vi "Error - Fire.vi"(6 "Data":variant, 8 "error in (no error)":errorcluster, 9 "Error Source":T1, 10 "Error Type":T2, 11 "View Model":T3) -> (0 "error out":errorcluster, 3 "View Model":T3)   [LabVIEW 2017]
doc: "Generate user Event for Error event"
uses:
  View Model/Controls/View Model.ctl
  View Model/Controls/Shared Model.ctl
  Controls/Error Model.ctl
  Controls/Error Data.ctl
  Controls/Error Type.ctl
  Controls/Error Source.ctl
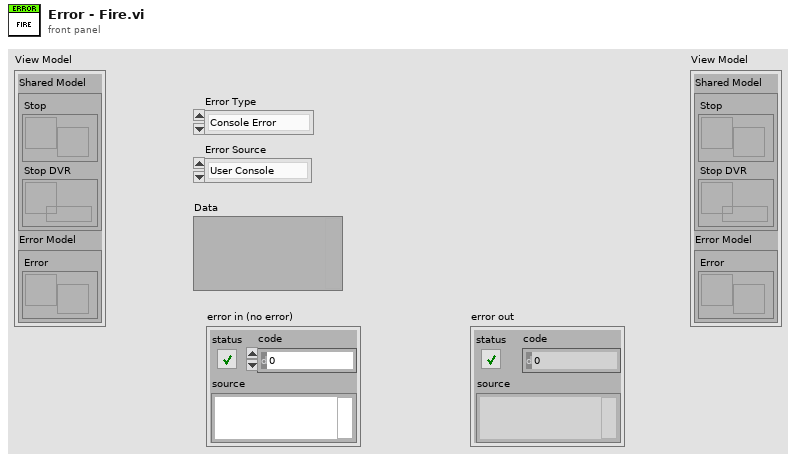
[diagram p1: front panel]
types:
  T1 = typedef "Error Source.ctl" = enum16{"User Console", "Display Console", "Sensor Interface"}
  T2 = typedef "Error Type.ctl" = enum16{"Console Error", "Sensor Interface IO Error", "Process Step Error"}
  T3 = typedef "View Model.ctl" = cluster{"Shared Model":T4, "Error Model":T5}
  T4 = typedef "Shared Model.ctl" = cluster{"Stop":refnum<user-event>, "Stop DVR":refnum<data-value>}
  T5 = typedef "Error Model.ctl" = cluster{"Error":refnum<user-event>}
  T6 = typedef "Error Data.ctl" = cluster{"Error Type":T2, "Error Source":T1, "Data":variant}
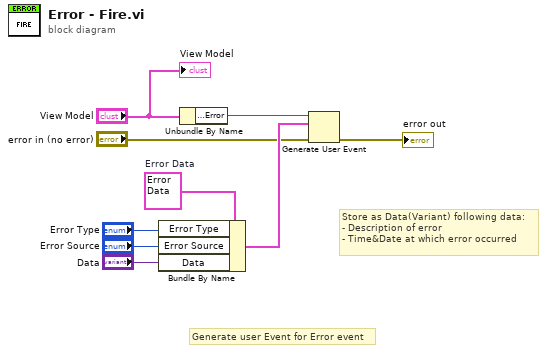
[diagram p0: block diagram]
diagram:
  w8 = T6 {"Error Type"=enum."Console Error", "Error Source"=enum."User Console", "Data"=variant}  # Error Data
  # "Store as Data(Variant) following data:\n- Description of error\n- Time&Date at which error occurred"
  # "Generate user Event for Error event"
  n1 = Bundle By Name(cluster=w8, "Error Type"="Error Type", "Error Source"="Error Source", "Data"="Data") -> (w7:T6)
  n2 = Unbundle By Name("View Model") -> ("Error Model.Error"=w9:refnum<user-event>)
  n3 = Generate User Event(user event=w9, event data cluster=w7, error in="error in (no error)") -> (error out=→"error out":errorcluster)  [unwired: 1 in, 1 out]
  "View Model" <- "View Model"
